vi "Do.vi"(8 "error in (no error)":errorcluster, 10 "Actor in":refnum<class "Actor.lvclass">, 11 "Update Fan Status Msg":refnum<class "Cooler Update Fan Status Msg.lvclass">) -> (0 "error out":errorcluster, 2 "Actor out":refnum<class "Actor.lvclass">)   [LabVIEW 2025, in "Evaporative Cooler.lvlib" / "Cooler Update Fan Status Msg.lvclass"]
uses:
  Cooler Update Fan Status Msg.lvclass
  <vilib>/ActorFramework/Actor/Actor.lvclass
  Evaporative Cooler/Evaporative Cooler.lvclass
  Dual Fan/Update Fan Status Msg/Update Fan Status Msg.lvclass/Update Fan Status Msg.ctl
  Cooler Update Fan Status Msg.lvclass/Cooler Update Fan Status Msg.ctl
  Dual Fan/Update Fan Status Msg/Update Fan Status Msg.lvclass
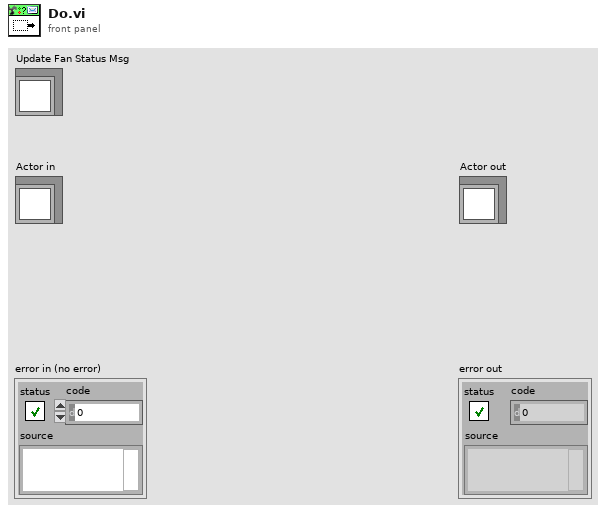
[diagram p1: front panel]
types:
  T1 = typedef "Dual Fan.lvlib/Dual Fan.lvclass/Fan Info.ctl" = cluster{"State":bool, "Fault":bool}
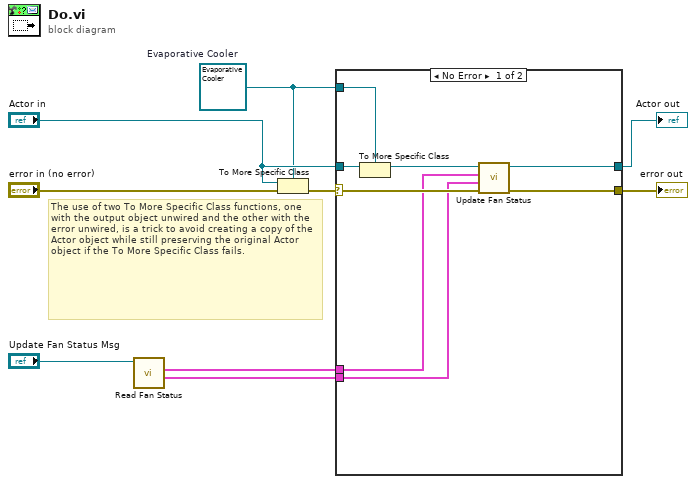
[diagram p0: block diagram]
diagram:
  w4 = refnum<class "Evaporative Cooler.lvclass"> refnum  # Evaporative Cooler
  # "The use of two To More Specific Class functions, one with the output object unwired and the other with the error unwired, is a trick to avoid creating a copy of the Actor object while still preserving the original Actor object if the To More Specific Class fails."
  n1 = call "Read Fan Status.vi"("Update Fan Status Msg in"="Update Fan Status Msg") -> ("Fan B"=w1:T1, "Fan A"=w2:T1)  [unwired: 9 in]
  n2 = To More Specific Class(target class=w4, reference="Actor in", error in="error in (no error)") -> (error out=w8:errorcluster)  [unwired: 1 out]
  n3 = case shown="No Error" w8 {
    selector: w8 -> [w15 w19]
    tunnel: [w17 w19] -> w7
    tunnel: [w16 w18] -> w6
    tunnel: "Actor in" -> [w14 w18]
    tunnel: w4 -> [w13 _]
    tunnel: w2 -> [w11 _]
    tunnel: w1 -> [w10 _]
    frame No Error {
      n4 = To More Specific Class(target class=w13, reference=w14) -> (specific class reference=w12:refnum<class "Evaporative Cooler.lvclass">)  [unwired: 1 in, 1 out]
      n5 = call-dynamic "Update Fan Status.vi"("error in (no error)"=w15, "Fan B"=w10, "Fan A"=w11, "Evaporative Cooler"=w12) -> ("error out"=w17:errorcluster, "Evaporative Cooler"=w16:refnum<class "Evaporative Cooler.lvclass">)  [unwired: 6 in]
    }
    frame Error {
      # "If type check fails, pass the original object out again."
    }
  }
  "error out" <- w7
  "Actor out" <- w6
